vi "Read.vi"(8 "error in (no error)":errorcluster, 11 "AI Ref In":T1) -> (0 "error out":errorcluster, 2 "Values":dbl[](array[numeric]), 3 "AI Ref Out":T1)   [LabVIEW 2021, in "AI.lvlib"]
doc: "Reads values from one or more analog input channels."
uses:
  <vilib>/myRIO/Instrument Drivers/Onboard IO/AI/AI.lvlib
  <vilib>/myRIO/Instrument Drivers/Onboard IO/AI/typedefs/AI Reference.ctl
  <vilib>/myRIO/Common/Instrument Driver Framework/Utilities/typedefs/myRIO Generic Hardware Reference.ctl
  <vilib>/myRIO/Common/Instrument Driver Framework/Utilities/typedefs/Hardware Version Enum.ctl
  <vilib>/myRIO/Common/Instrument Driver Framework/Utilities/typedefs/myRIO v1.0 Reference.ctl
  <vilib>/myRIO/Common/Instrument Driver Framework/Utilities/typedefs/Generic FPGA Reference.ctl
  <vilib>/myRIO/Common/Instrument Driver Framework/myRIO v1.0/AI/typedefs/AI Channels List.ctl
  <vilib>/myRIO/Common/Instrument Driver Framework/myRIO v1.0/AI/typedefs/AI Channels Enum.ctl
  <vilib>/myRIO/Common/Instrument Driver Framework/Utilities/typedefs/Analog Scaling Constants List.ctl
  <vilib>/myRIO/Common/Instrument Driver Framework/Utilities/typedefs/Analog Scaling Constants.ctl
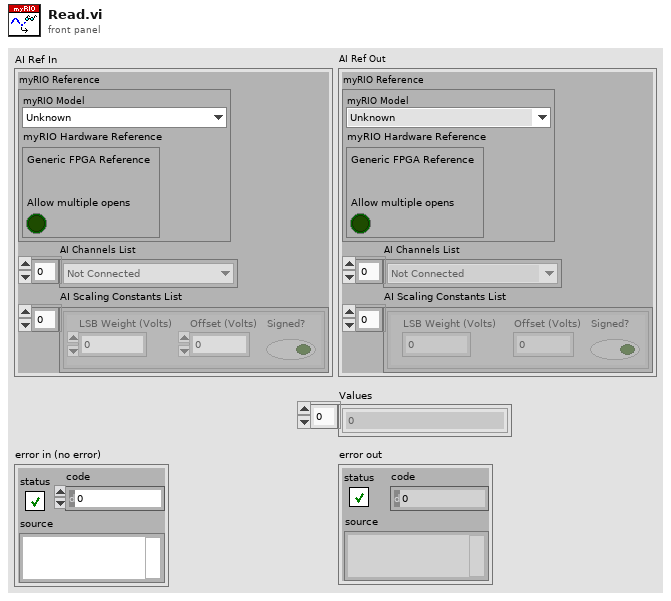
[diagram p1: front panel]
types:
  T1 = typedef "AI.lvlib/AI Reference.ctl" = cluster{"myRIO Reference":T2, "AI Channels List":T6, "AI Scaling Constants List":T8}
  T2 = typedef "myRIO Generic Hardware Reference.ctl" = cluster{"myRIO Model":T3, "myRIO Hardware Reference":T4}
  T3 = typedef "Hardware Version Enum.ctl" = enum16{"Unknown", "myRIO-1900", "myRIO-1950", "roboRIO", "NI ELVIS RIO CM", "ELVIS III"}
  T4 = typedef "myRIO v1.0 Reference.ctl" = cluster{"Generic FPGA Reference":T5, "Allow multiple opens":bool}
  T5 = typedef "Generic FPGA Reference.ctl" = refnum<k20>
  T6 = typedef "AI Channels List.ctl" = T7[]
  T7 = typedef "AI Channels Enum.ctl" = enum16{"Not Connected", "AudioIn/Left", "AudioIn/Right", "C/AI0", "C/AI1", "A/AI0", "A/AI1", "A/AI2", "A/AI3", "A/AI4", "A/AI5", "A/AI6", "A/AI7", "B/AI0", "B/AI1", "B/AI2", "B/AI3", "B/AI4", "B/AI5", "B/AI6", "B/AI7", "AI/AI0", "AI/AI1", "AI/AI2", "AI/AI3", "A/AI0 (DIFF)", "A/AI1 (DIFF)", "A/AI2 (DIFF)", "A/AI3 (DIFF)", "B/AI0 (DIFF)", "B/AI1 (DIFF)", "B/AI2 (DIFF)", "B/AI3 (DIFF)"}
  T8 = typedef "Analog Scaling Constants List.ctl" = T9[]
  T9 = typedef "Analog Scaling Constants.ctl" = cluster{"LSB Weight (Volts)":dbl, "Offset (Volts)":dbl, "Signed?":bool}
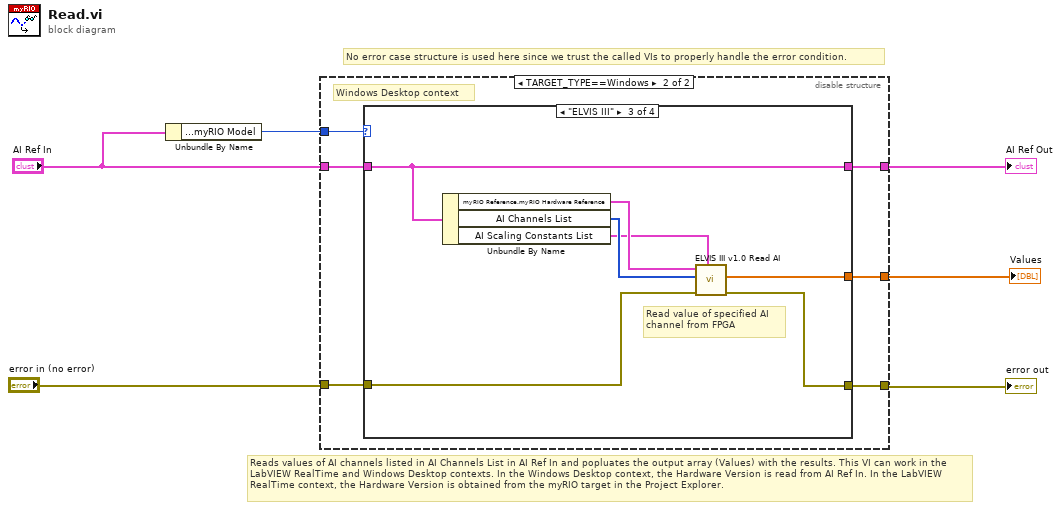
[diagram p0: block diagram]
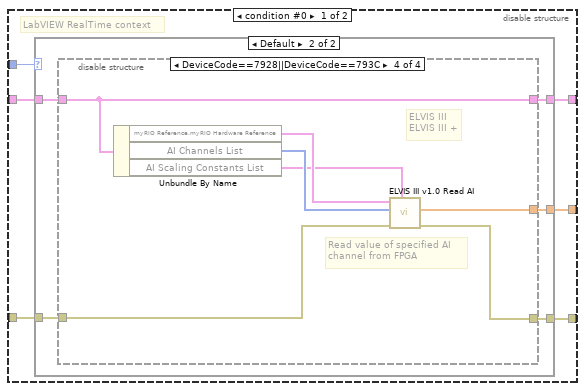
[diagram p2: hidden frame]
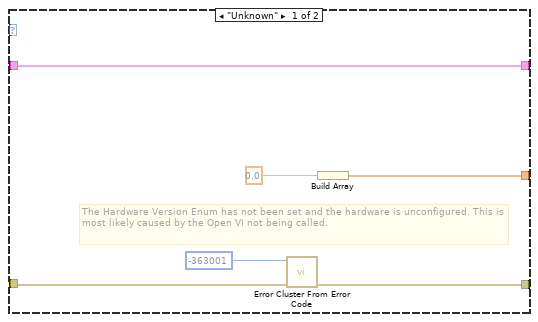
[diagram p3: hidden frame]
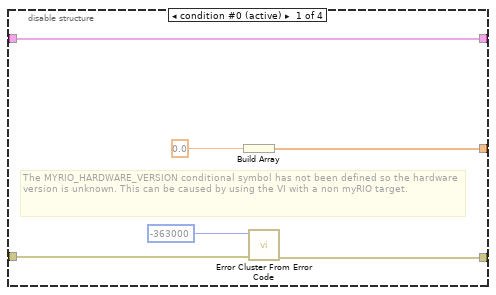
[diagram p4: hidden frame]
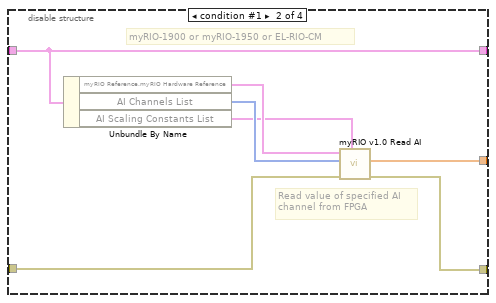
[diagram p5: hidden frame]
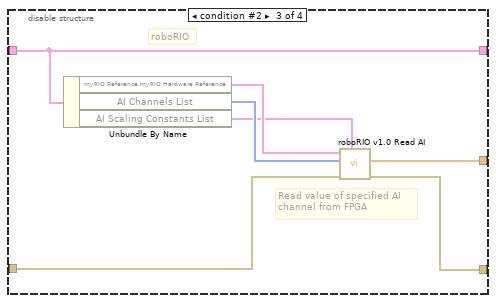
[diagram p6: hidden frame]
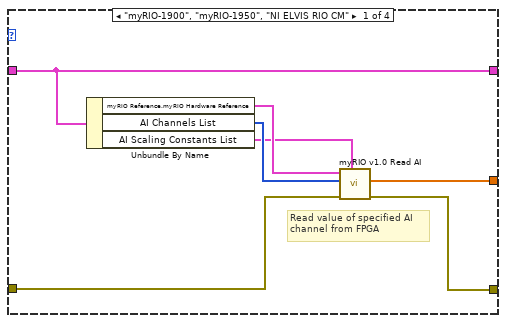
[diagram p7: hidden frame]
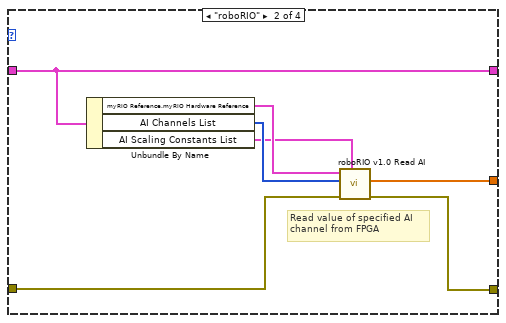
[diagram p8: hidden frame]
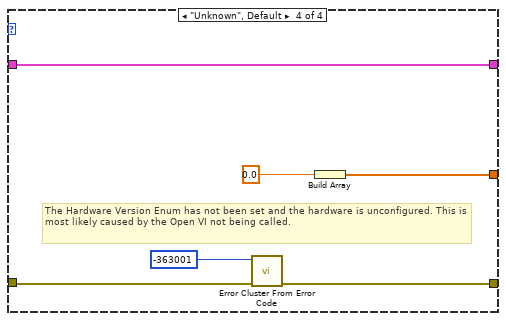
[diagram p9: hidden frame]
diagram:
  # "No error case structure is used here since we trust the called VIs to properly handle the error condition."
  # "Reads values of AI channels listed in AI Channels List in AI Ref In and popluates the output array (Values) with the results. This VI can work in the LabVIEW RealTime and Windows Desktop contexts. In the Windows Desktop context, the Hardware Version is read from AI Ref In. In the LabVIEW RealTime context, the Hardware Version is obtained from the myRIO target in the Project Explorer."
  n1 = Unbundle By Name("AI Ref In") -> ("myRIO Reference.myRIO Model"=w1:T3)
  n2 = disable-structure shown="TARGET_TYPE==Windows" {
    disable-tunnel: [w12 w56] -> w3
    disable-tunnel: "AI Ref In" -> [w11 w53]
    disable-tunnel: "error in (no error)" -> [w10 w55]
    disable-tunnel: [w9 w54] -> w4
    disable-tunnel: [w8 w52] -> w2
    disable-tunnel: w1 -> [w7 w51]
    frame condition #0 {
      # "LabVIEW RealTime context"
      n3 = case shown="Default" w7 {
        tunnel: [w15 w23] -> w12
        tunnel: w11 -> [w13 w22]
        tunnel: w10 -> [w16 w21]
        tunnel: [w13 w20] -> w9
        tunnel: [w14 w19] -> w8
        frame "Unknown" {
          # "The Hardware Version Enum has not been set and the hardware is unconfigured. This is most likely caused by the Open VI not being called."
          n4 = call <vilib>:"Error Cluster From Error Code.vi"("error in (no error)"=w16, "error code (0)"=-363001) -> ("error out"=w15:errorcluster)  [unwired: 7 in]
          n5 = Build Array(0.0 ("dbl Scaled Value")) -> (w14:dbl[])
        }
        frame Default {
          n6 = disable-structure shown="DeviceCode==7928||DeviceCode==793C" {
            disable-tunnel: w22 -> [w26 w35 w42 w47]
            disable-tunnel: [w29 w31 w38 w45] -> w23
            disable-tunnel: [w24 w32 w39 w46] -> w19
            disable-tunnel: w21 -> [w27 w34 w41 w44]
            disable-tunnel: [w26 w35 w42 w47] -> w20
            frame condition #0 (active) {
              # "The MYRIO_HARDWARE_VERSION conditional symbol has not been defined so the hardware version is unknown. This can be caused by using the VI with a non myRIO target."
              n7 = Build Array(0.0 ("dbl Scaled Value")) -> (w24:dbl[])
              n8 = call <vilib>:"Error Cluster From Error Code.vi"("error in (no error)"=w27, "error code (0)"=-363000) -> ("error out"=w29:errorcluster)  [unwired: 7 in]
            }
            frame condition #1 {
              # "myRIO-1900 or myRIO-1950 or EL-RIO-CM"
              # "Read value of specified AI \nchannel from FPGA"
              n9 = Unbundle By Name(w35) -> ("myRIO Reference.myRIO Hardware Reference"=w36:T4, "AI Channels List"=w33:T6, "AI Scaling Constants List"=w30:T8)
              n10 = call <vilib>:"myRIO v1.0 Read AI.vi"("Scale Constants Array"=w30, "error in (no error)"=w34, "Channel List"=w33, "myRIO Ref In"=w36) -> ("error out"=w31:errorcluster, "dbl Scaled Value List"=w32:dbl[])  [unwired: 5 in, 1 out]
            }
            frame condition #2 {
              # "roboRIO"
              # "Read value of specified AI \nchannel from FPGA"
              n11 = Unbundle By Name(w42) -> ("myRIO Reference.myRIO Hardware Reference"=w43:T4, "AI Channels List"=w40:T6, "AI Scaling Constants List"=w37:T8)
              n12 = call <vilib>:"roboRIO v1.0 Read AI.vi"("Scale Constants Array"=w37, "error in (no error)"=w41, "Channel List"=w40, "myRIO Ref In"=w43) -> ("error out"=w38:errorcluster, "dbl Scaled Value List"=w39:dbl[])  [unwired: 5 in, 1 out]
            }
            frame condition #3 {
              # "ELVIS III\nELVIS III +"
              # "Read value of specified AI \nchannel from FPGA"
              n13 = Unbundle By Name(w47) -> ("myRIO Reference.myRIO Hardware Reference"=w50:T4, "AI Channels List"=w49:T6, "AI Scaling Constants List"=w48:T8)
              n14 = call <vilib>:"ELVIS III v1.0 Read AI.vi"("Scale Constants Array"=w48, "error in (no error)"=w44, "Channel List"=w49, "myRIO Ref In"=w50) -> ("error out"=w45:errorcluster, "dbl Scaled Value List"=w46:dbl[])  [unwired: 5 in, 1 out]
            }
          }
        }
      }
    }
    frame condition #1 (active) {
      # "Windows Desktop context"
      n15 = case shown="\"ELVIS III\"" w51 {
        tunnel: [w59 w66 w73 w83] -> w56
        tunnel: w53 -> [w63 w70 w71 w80]
        tunnel: w55 -> [w60 w67 w74 w81]
        tunnel: [w63 w70 w71 w80] -> w54
        tunnel: [w58 w65 w72 w78] -> w52
        frame "myRIO-1900", "myRIO-1950", "NI ELVIS RIO CM" {
          # "Read value of specified AI \nchannel from FPGA"
          n16 = Unbundle By Name(w63) -> ("myRIO Reference.myRIO Hardware Reference"=w62:T4, "AI Channels List"=w61:T6, "AI Scaling Constants List"=w57:T8)
          n17 = call <vilib>:"myRIO v1.0 Read AI.vi"("Scale Constants Array"=w57, "error in (no error)"=w60, "Channel List"=w61, "myRIO Ref In"=w62) -> ("error out"=w59:errorcluster, "dbl Scaled Value List"=w58:dbl[])  [unwired: 5 in, 1 out]
        }
        frame "roboRIO" {
          # "Read value of specified AI \nchannel from FPGA"
          n18 = Unbundle By Name(w70) -> ("myRIO Reference.myRIO Hardware Reference"=w69:T4, "AI Channels List"=w68:T6, "AI Scaling Constants List"=w64:T8)
          n19 = call <vilib>:"roboRIO v1.0 Read AI.vi"("Scale Constants Array"=w64, "error in (no error)"=w67, "Channel List"=w68, "myRIO Ref In"=w69) -> ("error out"=w66:errorcluster, "dbl Scaled Value List"=w65:dbl[])  [unwired: 5 in, 1 out]
        }
        frame "ELVIS III" {
          # "Read value of specified AI \nchannel from FPGA"
          n20 = Unbundle By Name(w71) -> ("myRIO Reference.myRIO Hardware Reference"=w77:T4, "AI Channels List"=w76:T6, "AI Scaling Constants List"=w75:T8)
          n21 = call <vilib>:"ELVIS III v1.0 Read AI.vi"("Scale Constants Array"=w75, "error in (no error)"=w74, "Channel List"=w76, "myRIO Ref In"=w77) -> ("error out"=w73:errorcluster, "dbl Scaled Value List"=w72:dbl[])  [unwired: 5 in, 1 out]
        }
        frame "Unknown", Default {
          # "The Hardware Version Enum has not been set and the hardware is unconfigured. This is most likely caused by the Open VI not being called."
          n22 = call <vilib>:"Error Cluster From Error Code.vi"("error in (no error)"=w81, "error code (0)"=-363001) -> ("error out"=w83:errorcluster)  [unwired: 7 in]
          n23 = Build Array(0.0 ("dbl Scaled Value")) -> (w78:dbl[])
        }
      }
    }
  }
  "AI Ref Out" <- w4
  "error out" <- w3
  "Values" <- w2
